vi "Get DescentPoint.vi"(8 "error in (no error)":errorcluster, 9 "Character type":T1=enum."ASCII", 10 "Font refnum":refnum<k24>, 11 "String":string) -> (0 "error out":errorcluster, 3 "DescentPoint":sgl)   [LabVIEW 2020, in "Exaprom PDF.lvlib" / "Font Class.lvclass"]
doc: "Version 2.0\nDeveloped by Jean-Marc Simard\nCopyright © 2012, Exaprom Inc.\nAll rights reserved.\nLicense: BSD\n\nWith iTextSharp 4.1.6 (http://itextsharp.sourceforge.net)\nunder Mozilla Public License Version 1.1\n(http://www.mozilla.org/MPL/MPL-1.1.html)"
uses:
  <userlib>/labview-PDF-writer-master/LV Class/Fonts Class/Font Class.lvclass
  C:/Program Files (x86)/National Instruments/LabVIEW 2020/user.lib/labview-PDF-writer-master/DLL/itextsharp.dll
  DLL/itextsharp.dll
  <userlib>/labview-PDF-writer-master/Controls/Text Controls/Unicode/Type and run direction.ctl
  <userlib>/labview-PDF-writer-master/Exaprom PDF.lvlib
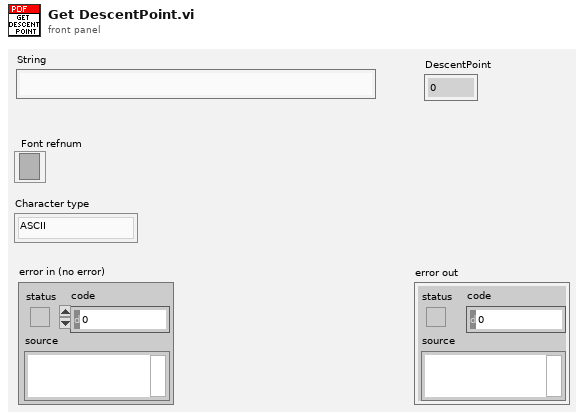
[diagram p1: front panel]
types:
  T1 = typedef "Exaprom PDF.lvlib/Type and run direction.ctl" = enum16{"Select", "ASCII", "UTF-16", "UTF-16 (default)", "UTF-16 (LTR)", "UTF-16 (RTL)"}
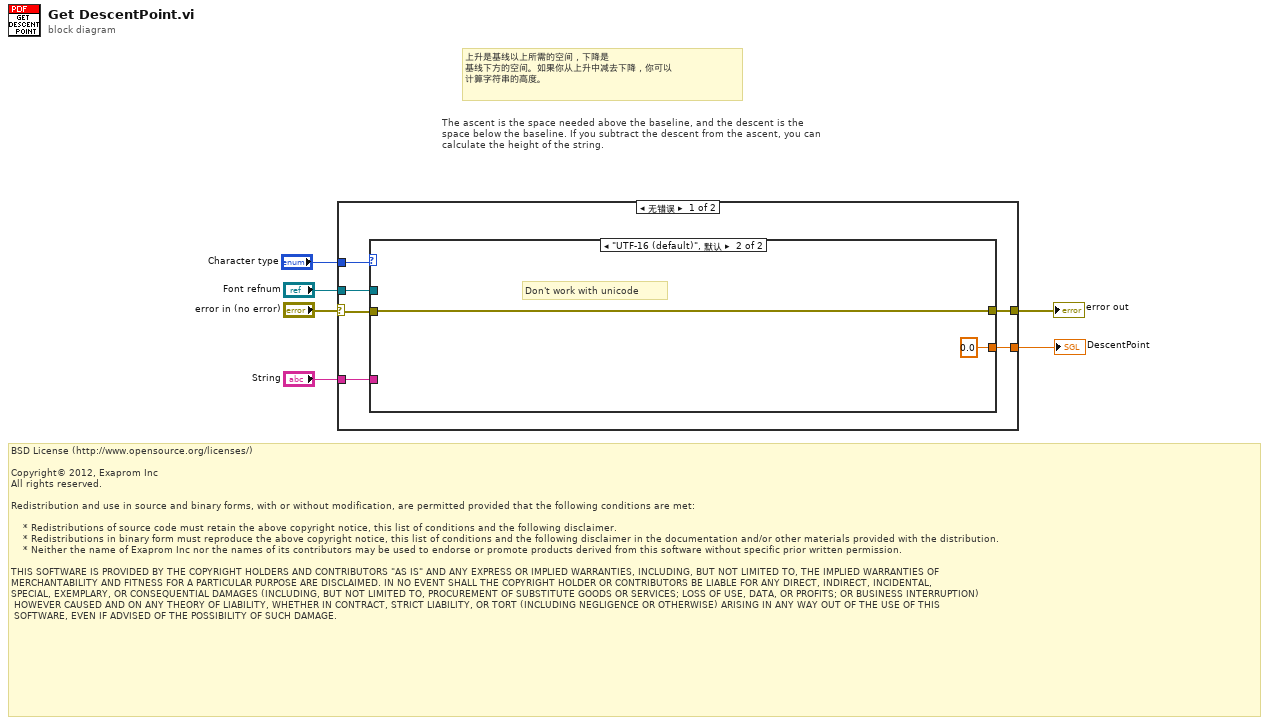
[diagram p0: block diagram]
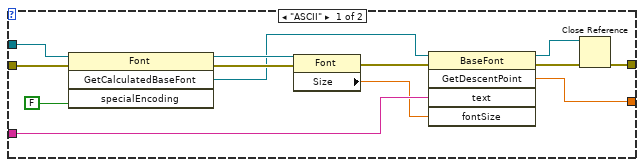
[diagram p2: hidden frame]
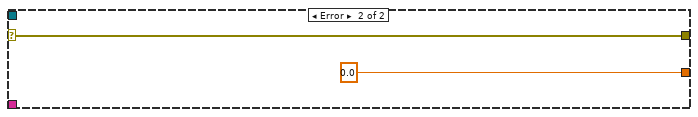
[diagram p3: hidden frame]
diagram:
  # "上升是基线以上所需的空间，下降是\n基线下方的空间。如果你从上升中减去下降，你可以\n计算字符串的高度。"
  # "The ascent is the space needed above the baseline, and the descent is the\nspace below the baseline. If you subtract the descent from the ascent, you can\ncalculate the height of the string."
  # "BSD License (http://www.opensource.org/licenses/)\n\nCopyright© 2012, Exaprom Inc\nAll rights reserved.\n\nRedistribution and use in source and binary forms, with or without modification, are permitted provided that the following conditions are met:\n\n    * Redistributions of source code must retain the above copyright notice, this list of conditions and the following disclaimer.\n    * Redistributions in binary form must reproduce the above copyright notice, this list of conditions and the following disclaimer in the documentation and/or other materials provided with the distribution.\n    * Neither the name of Exaprom Inc nor the names of its contributors may be used to endorse or promote products derived from this software without specific prior written permission.\n\nTHIS SOFTWARE IS PROVIDED BY THE COPYRIGHT HOLDERS AND CONTRIBUTORS \"AS IS\" AND ANY EXPRESS OR IMPLIED WARRANTIES, INCLUDING, BUT NOT LIMITED TO, THE IMPLIED WARRANTIES OF \nMERCHANTABILITY AND FITNESS FOR A PARTICULAR PURPOSE ARE DISCLAIMED. IN NO EVENT SHALL THE COPYRIGHT HOLDER OR CONTRIBUTORS BE LIABLE FOR ANY DIRECT, INDIRECT, INCIDENTAL,\nSPECIAL, EXEMPLARY, OR CONSEQUENTIAL DAMAGES (INCLUDING, BUT NOT LIMITED TO, PROCUREMENT OF SUBSTITUTE GOODS OR SERVICES; LOSS OF USE, DATA, OR PROFITS; OR BUSINESS INTERRUPTION)\n HOWEVER CAUSED AND ON ANY THEORY OF LIABILITY, WHETHER IN CONTRACT, STRICT LIABILITY, OR TORT (INCLUDING NEGLIGENCE OR OTHERWISE) ARISING IN ANY WAY OUT OF THE USE OF THIS\n SOFTWARE, EVEN IF ADVISED OF THE POSSIBILITY OF SUCH DAMAGE."
  n1 = case shown="无错误" "error in (no error)" {
    selector: "error in (no error)" -> [w9 w29]
    tunnel: "String" -> [w12 _]
    tunnel: [w8 w29] -> w5
    tunnel: [w11 sgl 0.0 ("GetDescentPoint")] -> w3
    tunnel: "Font refnum" -> [w10 _]
    tunnel: "Character type" -> [w7 _]
    frame No Error {
      n2 = case shown="\"UTF-16 (default)\", 默认" w7 {
        tunnel: w12 -> [w24 _]
        tunnel: [w23 sgl 0.0 ("GetDescentPoint")] -> w11
        tunnel: w10 -> [w22 _]
        tunnel: w9 -> [w21 w27]
        tunnel: [w16 w27] -> w8
        frame "ASCII" {
          n3 = invoke class="Font" method="GetCalculatedBaseFont"(reference=w22, error in=w21, "specialEncoding"=FALSE) -> (reference out=w14:refnum<k24>, error out=w20:errorcluster, "GetCalculatedBaseFont"=w13:refnum<k24>)  [unwired: 1 in, 1 out]
          n4 = property class="Font"(reference=w14, error in=w20) -> (error out=w18:errorcluster, "Size"=w19:sgl)  [unwired: 1 out]
          n5 = invoke class="BaseFont" method="GetDescentPoint"(reference=w13, error in=w18, "text"=w24, "fontSize"=w19) -> (reference out=w15:refnum<k24>, error out=w17:errorcluster, "GetDescentPoint"=w23:sgl)  [unwired: 1 in, 2 out]
          n6 = Close Reference(reference=w15, error in (no error)=w17) -> (error out=w16:errorcluster)
        }
        frame "UTF-16 (default)", Default {
          # "Don't work with unicode"
        }
      }
    }
    frame Error {
    }
  }
  "error out" <- w5
  "DescentPoint" <- w3
